vi "logg.vi"() -> ()   [LabVIEW 2010]
uses:
  <vilib>/Platform/TimedLoop/XDataNode/nitl_modes.ctl
  <vilib>/Platform/TimedLoop/XDataNode/XDataNode.xnode
  <vilib>/Platform/TimedLoop/XDataNode/timing_clust.ctl
  <vilib>/Platform/TimedLoop/XDataNode/wakeup.ctl
  <vilib>/Platform/TimedLoop/XDataNode/XDNodeRunTimeDep.lvlib
panel:
  out "Elapsed Time [s]":dbl
  out "Sample #":dbl
  in  "stop":bool
  out "Write to file":string
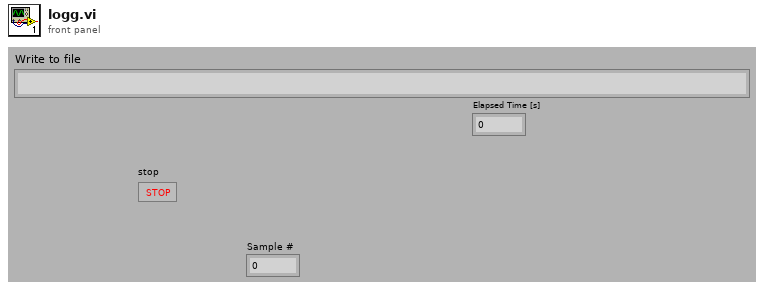
[diagram p1: front panel]
types:
  T1 = enum16{"open", "replace", "create", "open or create", "replace or create", "replace or create with confirmation"}
  T2 = typedef "XDNodeRunTimeDep.lvlib/timing_clust.ctl" = cluster{"Expected End [f-1]":u64, "Actual End [f-1]":u64, "Finished Late? [f-1]":bool, "Expected End [i-1]":u64, "Actual End [i-1]":u64, "Finished Late? [i-1]":bool, "Expected Start [i]":u64, "Actual Start [i]":u64, "Expected Start [f]":u64, "Actual Start [f]":u64, "Source Name":string, "Structure Name":string, "Period":i64, "Deadline":i64, "Offset":i64, "Start":i64, "Priority":i32, "Timeout":i32, "Mode":T3, "Wakeup Reason":T4, "Error":errorcluster, "Source Type":string, "Secondary Source Type":string, "Global End Time":u64, "Global Start Time":u64, "Frame Duration":u64, "Iteration Duration":u64, "Assigned CPU":i32, "I/O Scan Engine Mode":u32}
  T3 = typedef "XDNodeRunTimeDep.lvlib/nitl_modes.ctl" = enum32{"No Change", "Process missed periods, maintain original phase", "Discard missed periods, maintain original phase", "Process missed periods, ignore original phase", "Discard missed periods, ignore original phase"}
  T4 = typedef "XDNodeRunTimeDep.lvlib/wakeup.ctl" = enum32{"Normal", "Aborted", "Asynchronous wakeup", "Timing source error", "Timed loop error", "Timeout"}
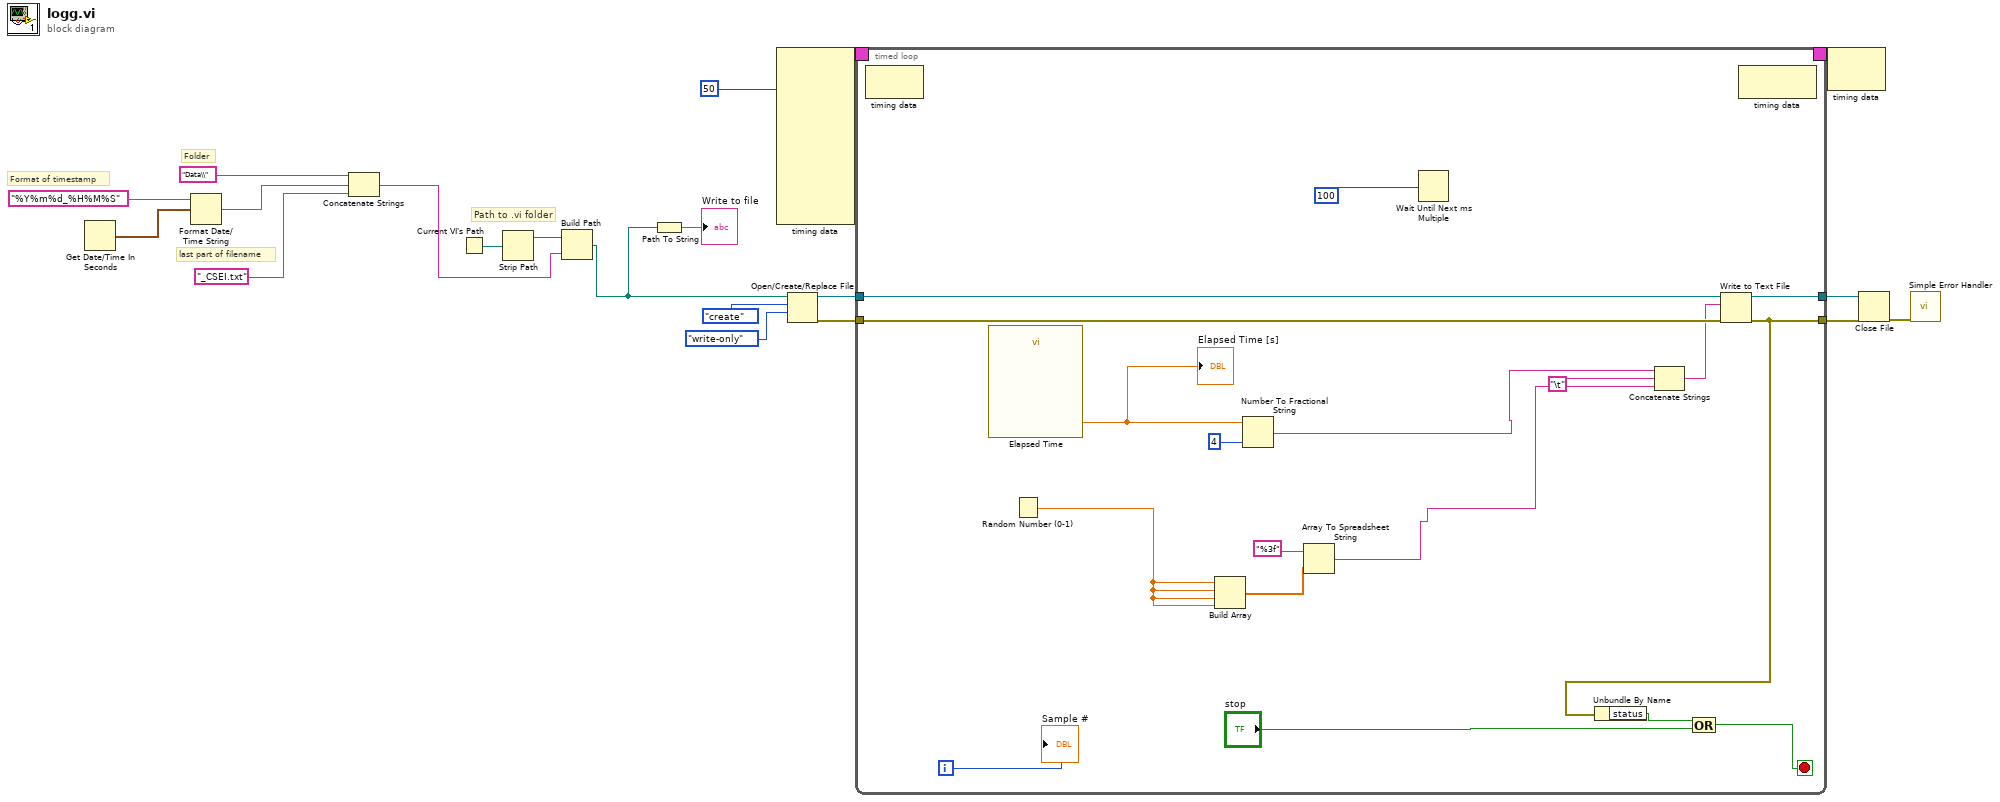
[diagram p0: block diagram]
diagram:
  # "Path to .vi folder"
  # "last part of filename"
  # "Folder"
  # "Format of timestamp"
  n1 = Get Date/Time In Seconds() -> (seconds since 1Jan1904=w19:timestamp)
  n2 = Format Date/Time String(time format string (%c)="%Y%m%d_%H%M%S", seconds (now)=w19) -> (date/time string=w17:string)  [unwired: 1 out]
  n3 = Concatenate Strings("Data\\" ("string"), w17, "_CSEI.txt" ("string")) -> (w13:string)
  n4 = Current VI's Path() -> (path=w16:path)
  n5 = Strip Path(path=w16) -> (stripped path=w15:path)  [unwired: 1 out]
  n6 = Build Path(base path=w15, name or relative path=w13) -> (appended path=w7:path)
  n7 = Path To String(path=w7) -> (string=→"Write to file":string)
  n8 = node-c288(50) -> (w11:T2)  [unwired: 9 in]
  n9 = Open/Create/Replace File(file path (use dialog)=w7, operation (0:open)=T1."create", access (0:read/write)=enum16{"read/write", "read-only", "write-only"}."write-only") -> (refnum out=w6:refnum<file>, error out=w4:errorcluster)  [unwired: 3 in, 1 out]
  n10 = timed-loop {
    timing: w11 -> [_]
    timing-out: [_] -> w10
    tunnel: w6 -> [w38]
    tunnel: [w37] -> w5
    tunnel: w4 -> [w36]
    tunnel: [w24] -> w3
    i -> [w31]
    stop <- w23 stop-if-true
    n11 = node-c288() -> ()  [unwired: 1 in, 1 out]
    n12 = call "Elapsed Time"() -> ("Elapsed Time (s)"=w25:dbl)  [unwired: 12 in, 7 out]
    "Elapsed Time [s]" <- w25
    n13 = Random Number (0-1)() -> (number: 0 to 1=w27:dbl)
    n14 = Build Array(w27, w27, w27, w27) -> (w28:dbl[])
    n15 = Number To Fractional String(number=w25, precision (6)=4) -> (F-format string=w32:string)  [unwired: 2 in]
    n16 = Array To Spreadsheet String(array=w28, 3:"%3f") -> (spreadsheet string=w26:string)  [unwired: 1 in]
    n17 = Wait Until Next ms Multiple(millisecond multiple=100) -> ()  [unwired: 1 out]
    n18 = Concatenate Strings(w32, "\t", w26) -> (w35:string)
    n19 = Write to Text File(file (use dialog)=w38, text=w35, error in=w36) -> (refnum out=w37:refnum<file>, error out=w24:errorcluster)  [unwired: 1 in, 1 out]
    n20 = Unbundle By Name(w24) -> ("status"=w21:bool)
    n21 = Compound Arithmetic op=OR(w21, "stop") -> (w23:bool)
    n22 = node-c288() -> ()  [unwired: 1 in, 1 out]
    "Sample #" <- w31
  }
  n23 = node-c288(w10) -> ()  [unwired: 1 out]
  n24 = Close File(refnum=w5, error in=w3) -> (error out=w2:errorcluster)  [unwired: 1 out]
  n25 = call <vilib>:"Simple Error Handler.vi"("error in (no error)"=w2) -> ()  [unwired: 4 in, 5 out]
